vi "Real pool navigation1.vi"() -> ()   [LabVIEW 2011]
uses:
  <vilib>/userdefined/High Color/IMAQdx.ctl
  <vilib>/vision/driver/NI_Vision_Acquisition_Software.lvlib
panel:
  in  "stop":bool
  in  "Session In":T1="cam2"
  out "Whale":cluster{"x":sgl, "y":sgl}
  out "Bouy":cluster{"x":sgl, "y":sgl}
  out "Boat":cluster{"x":sgl, "y":sgl}
  out "Boat\nHeading":sgl
  out "Location":cluster{"x":sgl, "y":sgl}
  out "error out":errorcluster
  out "Pool Image":T2(plugin-control)
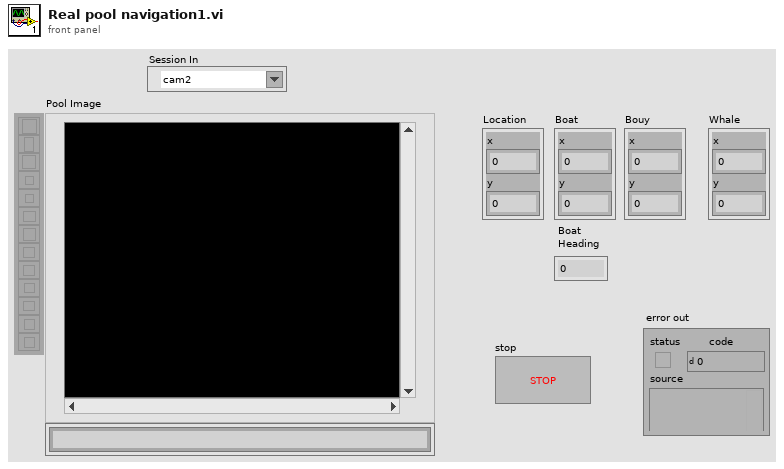
[diagram p1: front panel]
types:
  T1 = typedef "IMAQdx.ctl" = refnum<k21>
  T2 = typedef "IMAQ Image.ctl" = refnum<image>
  T3 = typedef "Image Type" = u32
  T4 = typedef "IMAQ GM Match Report.ctl" = cluster{"Position":cluster{"x":sgl, "y":sgl}, "Angle":sgl, "Scale":sgl, "Score":sgl, "Bounding Box":cluster{"x":sgl, "y":sgl}[], "Contrast Reversed":bool, "Occlusion %":sgl, "Template Target Curve Score":sgl, "Target Template Curve Score":sgl, "Correlation Score":sgl}
  T5 = cluster{"Position":cluster{"x":sgl, "y":sgl}, "Angle":sgl, "Scale":sgl, "Score":sgl, "Bounding Box":cluster{"x":sgl, "y":sgl}[]}[]
  T6 = cluster{"Position":cluster{"x":sgl, "y":sgl}, "Angle":sgl, "Scale":sgl, "Score":sgl, "Bounding Box":cluster{"x":sgl, "y":sgl}[]}
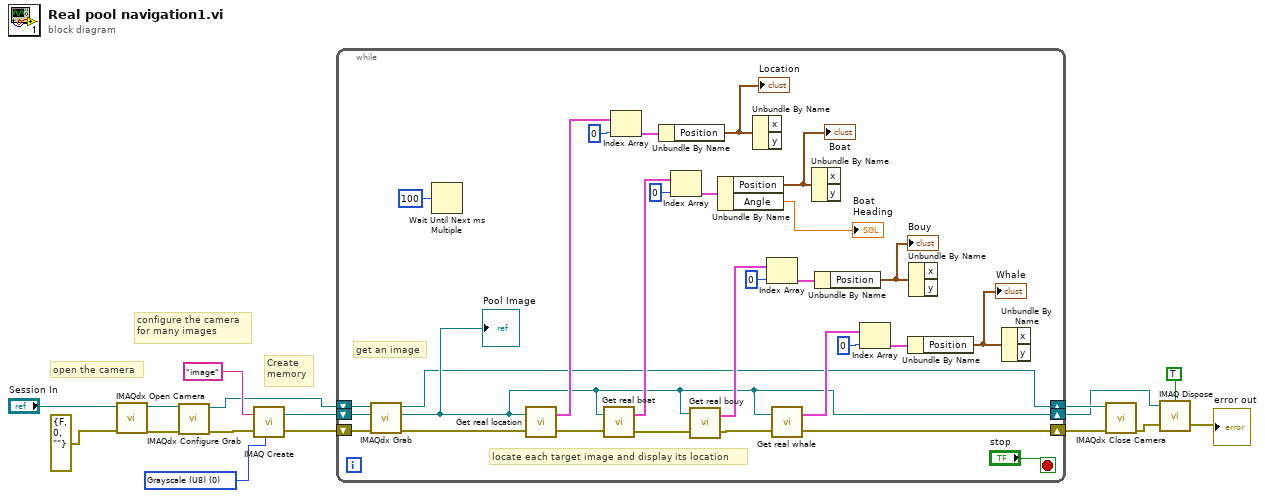
[diagram p0: block diagram]
diagram:
  w14 = T3 0 items=["Grayscale (U8)", "Grayscale (I16)", "Grayscale (SGL)", "Complex (CSG)", "RGB (U32)", "HSL (U32)", "RGB (U64)", "Grayscale (U16)"] ("Image Type")
  # "Create \nmemory"
  # "configure the camera\nfor many images"
  # "open the camera"
  n1 = call <vilib>:"IMAQdx Open Camera.vi"("error in"=errorcluster {"status"=FALSE, "code"=0, "source"=""} ("error in (no error)"), "Session In"="Session In") -> ("error out"=w13:errorcluster, "Session Out"=w11:T1)  [unwired: 1 in, 7 out]
  n2 = call <vilib>:"IMAQdx Configure Grab.vi"("error in"=w13, "Session In"=w11) -> ("error out"=w12:errorcluster, "Session Out"=w6:T1)  [unwired: 8 out]
  n3 = call "IMAQ Create"("Image Name"="image", "Image Type"=w14, "error in (no error)"=w12) -> ("New Image"=w5:T2, "error out"=w7:errorcluster)  [unwired: 1 in, 1 out]
  n4 = while {
    shift-right: [w19] -> w3
    shift-left: w6 -> [w24]
    shift-right: [w20] -> w1
    shift-left: w5 -> [w23]
    shift-right: [w21] -> w4
    shift-left: w7 -> [w25]
    stop <- "stop" stop-if-true
    # "locate each target image and display its location"
    # "get an image"
    n5 = call <vilib>:"IMAQdx Grab.vi"("error in"=w25, "Image In"=w23, "Session In"=w24) -> ("error out"=w22:errorcluster, "Image Out"=w20:T2, "Session Out"=w19:T1)  [unwired: 1 in, 5 out]
    "Pool Image" <- w20
    n6 = Wait Until Next ms Multiple(millisecond multiple=u32 100) -> ()  [unwired: 1 out]
    n7 = call "Get real location.vi"("error in"=w22, "Image"=w20) -> ("error out"=w42:errorcluster, "Matches"=w43:T4[])
    n8 = call "Get real boat.vi"("error in"=w42, "Image"=w20) -> ("error out"=w35:errorcluster, "Matches"=w36:T4[])
    n9 = Index Array(array=w43, index=0) -> (element=w45:T4)
    n10 = Unbundle By Name(w45) -> ("Position"=w44:cluster{"x":sgl, "y":sgl})
    "Location" <- w44
    n11 = Index Array(array=w36, index=0) -> (element=w40:T4)
    n12 = call "Get real bouy.vi"("error in"=w35, "Image"=w20) -> ("error out"=w30:errorcluster, "Matches"=w31:T4[])
    n13 = Unbundle By Name(w40) -> ("Position"=w39:cluster{"x":sgl, "y":sgl}, "Angle"=→"Boat\nHeading":sgl)
    "Boat" <- w39
    n14 = Unbundle By Name(w44) -> ()  [unwired: 2 out]
    n15 = Index Array(array=w31, index=0) -> (element=w33:T4)
    n16 = call "Get real whale.vi"("error in"=w30, "Image"=w20) -> ("error out"=w21:errorcluster, "Matches"=w26:T5)
    n17 = Unbundle By Name(w39) -> ()  [unwired: 2 out]
    n18 = Unbundle By Name(w33) -> ("Position"=w32:cluster{"x":sgl, "y":sgl})
    "Bouy" <- w32
    n19 = Index Array(array=w26, index=0) -> (element=w29:T6)
    n20 = Unbundle By Name(w29) -> ("Position"=w28:cluster{"x":sgl, "y":sgl})
    "Whale" <- w28
    n21 = Unbundle By Name(w32) -> ()  [unwired: 2 out]
    n22 = Unbundle By Name(w28) -> ()  [unwired: 2 out]
  }
  n23 = call <vilib>:"IMAQdx Close Camera.vi"("error in"=w4, "Session In"=w3) -> ("error out"=w2:errorcluster)  [unwired: 9 out]
  n24 = call "IMAQ Dispose"("All Images? (No)"=TRUE, "Image"=w1, "error in (no error)"=w2) -> ("error out"=→"error out":errorcluster)  [unwired: 3 in]
